vi "Read OPCUA Setting.vi"(8 "error in (no error)":errorcluster, 9 "Xml Filename":string, 10 "SubFolder In":string, 11 "Folder In":string) -> (0 "error out":errorcluster, 2 "OPCUA Setting Out":T1, 3 "OPCUA Path Out":path)   [LabVIEW 2024, in "OPCUA.lvlib"]
uses:
  OPCUA.lvlib
  OPCUA Setting.ctl
  <vilib>/Utility/xml.llb/Write to XML File(string).vi
  <vilib>/Utility/xml.llb/Read From XML File(string).vi
panel:
  in  "OPCUA":T1={"ServerName"="DataLogger", "Port"="49580", "Certificate File"=path "", "LDS URL"="opc.tcp://localhost:4840", "LDS Certificate File"=path "C:/ProgramData/OPC Foundation/UA/pki/own/certs/ualdscert.der", "Trust All Clients"=TRUE, "ClientConnect"="opc.tcp://localhost:49580", "NodeId"=""}
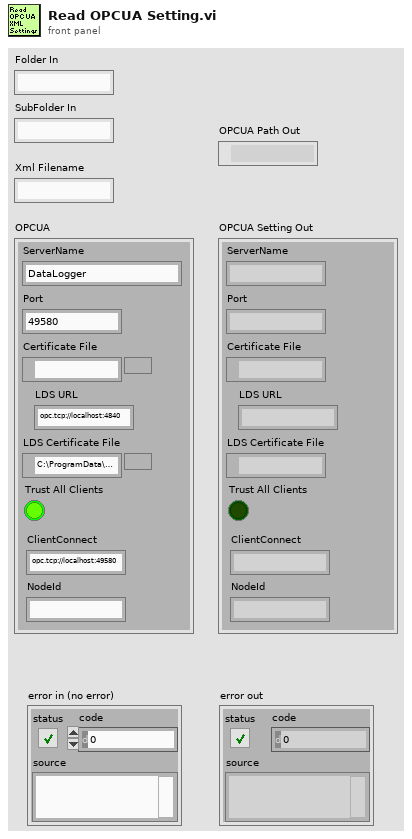
[diagram p1: front panel]
types:
  T1 = typedef "OPCUA.lvlib/OPCUA Setting.ctl" = cluster{"ServerName":string, "Port":string, "Certificate File":path, "LDS URL":string, "LDS Certificate File":path, "Trust All Clients":bool, "ClientConnect":string, "NodeId":string}
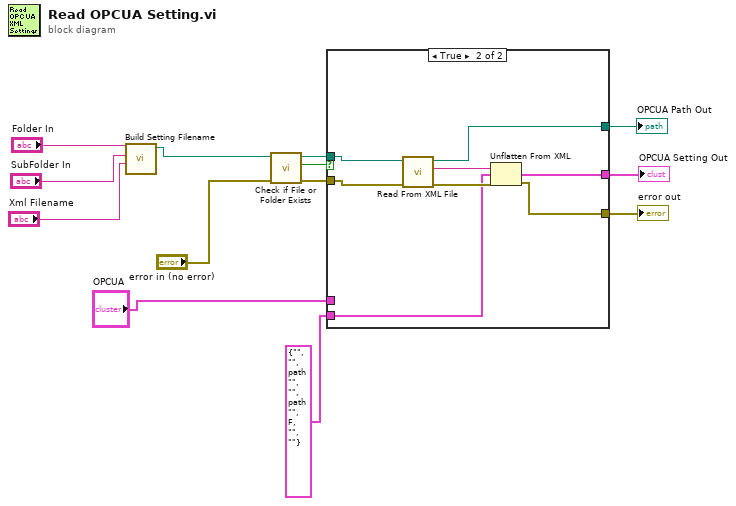
[diagram p0: block diagram]
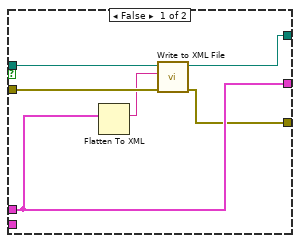
[diagram p2: hidden frame]
diagram:
  n1 = call "Build Setting Filename.vi"("Xml Filename In"="Xml Filename", "SubFolder In"="SubFolder In", "Folder In"="Folder In") -> ("Full Filename Out"=w1:path)  [unwired: 8 in]
  n2 = call <vilib>:"Check if File or Folder Exists.vi"("error in (no error)"="error in (no error)", "path"=w1) -> ("error out"=w11:errorcluster, "file or folder exists?"=w12:bool, "dup path"=w10:path)  [unwired: 7 in]
  n3 = case shown="True" w12 {
    tunnel: w11 -> [w17 w26]
    tunnel: w10 -> [w18 w27]
    tunnel: "OPCUA" -> [w19 _]
    tunnel: [w15 w23] -> w9
    tunnel: [w19 w20] -> w5
    tunnel: [w14 w22] -> w8
    tunnel: T1 {"ServerName"="", "Port"="", "Certificate File"=path "", "LDS URL"="", "LDS Certificate File"=path "", "Trust All Clients"=FALSE, "ClientConnect"="", "NodeId"=""} ("OPCUA Setting Out") -> [_ w21]
    frame False {
      n4 = Flatten To XML(6:w19) -> (2:w16:string)
      n5 = call-poly <vilib>:"Write to XML File.vi"("error in (no error)"=w17, "XML Input"=w16, "XML File Path"=w18) -> ("error out"=w14:errorcluster, "XML File Path(duplicate)"=w15:path)  [unwired: 6 in, 1 out]
    }
    frame True {
      n6 = call-poly <vilib>:"Read From XML File.vi"("error in (no error)"=w26, "XML File Path"=w27) -> ("error out"=w25:errorcluster, "XML Elements"=w24:string, "XML File Path(duplicate)"=w23:path)  [unwired: 7 in]
      n7 = Unflatten From XML(xml string=w24, type=w21, error in (no error)=w25) -> (value=w20:T1, error out=w22:errorcluster)
    }
  }
  "OPCUA Setting Out" <- w5
  "error out" <- w8
  "OPCUA Path Out" <- w9
